vi "Init.vi"(8 "error in (no error)":errorcluster, 10 "VMR":refnum<class "VMR.lvclass">) -> (0 "error out":errorcluster, 3 "ToggleMuteController out":refnum<class "ToggleMuteController.lvclass">)   [LabVIEW 2022 SP3, in "VMR-Deck.lvlib" / "ToggleMuteController.lvclass"]
uses:
  ToggleMuteController.lvclass
  ToggleMuteController.lvclass/ToggleMuteController.ctl
  VMR/VMR.lvclass
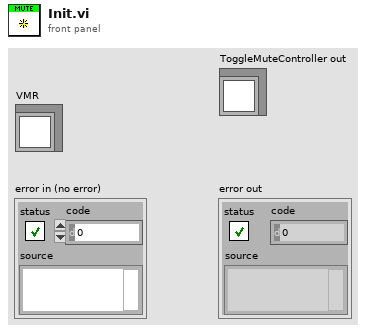
[diagram p1: front panel]
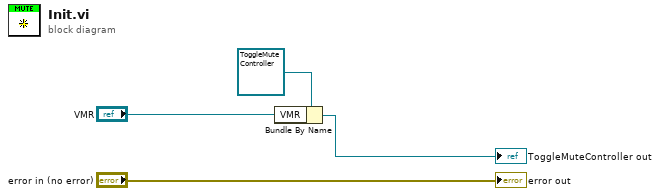
[diagram p0: block diagram]
diagram:
  n1 = Bundle By Name(cluster=refnum<class "ToggleMuteController.lvclass"> refnum ("ToggleMuteController in"), "VMR"="VMR") -> (→"ToggleMuteController out":refnum<class "ToggleMuteController.lvclass">)
  "error out" <- "error in (no error)"
